vi "Dispose.vi"(8 "error in (no error)":errorcluster, 11 "STOMP in":refnum<class "STOMP.lvclass">) -> (0 "error out":errorcluster, 3 "STOMP out":refnum<class "STOMP.lvclass">)   [LabVIEW 2017, in "LabVIEW STOMP.lvlib" / "STOMP.lvclass"]
uses:
  STOMP.lvclass
  STOMP.lvclass/STOMP.ctl
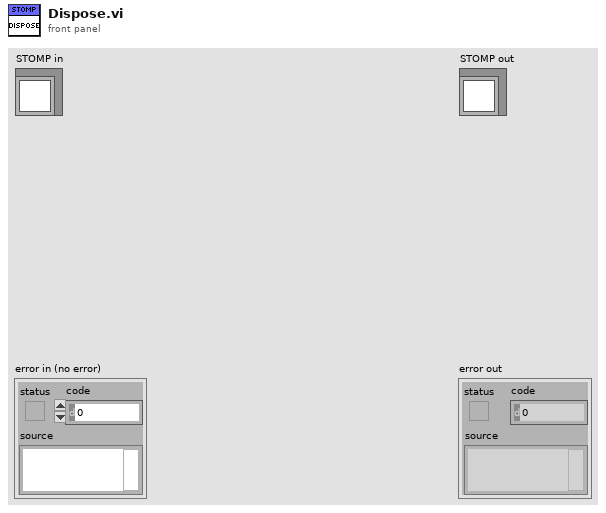
[diagram p1: front panel]
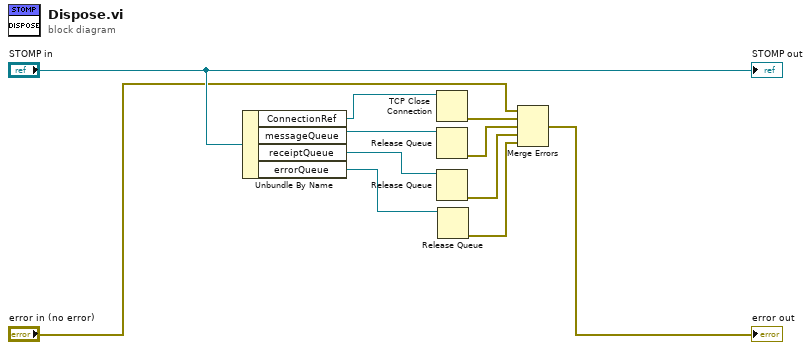
[diagram p0: block diagram]
diagram:
  n1 = Unbundle By Name("STOMP in") -> ("ConnectionRef"=w7:refnum<k5>, "messageQueue"=w9:refnum<queue>, "receiptQueue"=w8:refnum<queue>, "errorQueue"=w10:refnum<queue>)
  n2 = TCP Close Connection(connection ID=w7) -> (error out=w6:errorcluster)  [unwired: 2 in, 1 out]
  n3 = Release Queue(queue=w9) -> (error out=w5:errorcluster)  [unwired: 2 in, 2 out]
  n4 = Release Queue(queue=w8) -> (error out=w4:errorcluster)  [unwired: 2 in, 2 out]
  n5 = Release Queue(queue=w10) -> (error out=w3:errorcluster)  [unwired: 2 in, 2 out]
  n6 = Merge Errors("error in (no error)", w6, w5, w4, w3) -> (→"error out":errorcluster)
  "STOMP out" <- "STOMP in"
